vi "Draw Loops.vi"(7 "Action Diagram Sizing":T1, 10 "Action Diagram In":picture, 11 "Actions":T2={"Init"=FALSE, "Start"=FALSE, "Run"=TRUE, "Stop"=FALSE, "Close"=FALSE}) -> (2 "Action Diagram":picture)   [LabVIEW 2022 SP3, in "FlexBlocks Support.lvlib"]
uses:
  FlexBlocks Support.lvlib
  Action Selections.ctl
  Action Diagram Sizing.ctl
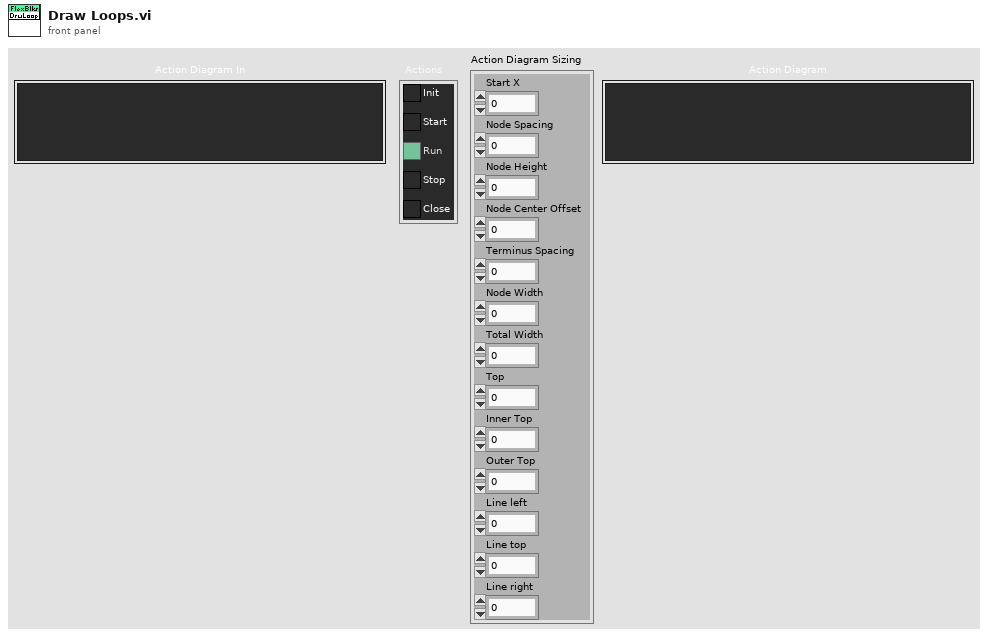
[diagram p1: front panel]
types:
  T1 = typedef "FlexBlocks Support.lvlib/Action Diagram Sizing.ctl" = cluster{"Start X":i32, "Node Spacing":i32, "Node Height":i32, "Node Center Offset":i32, "Terminus Spacing":i32, "Node Width":i32, "Total Width":i32, "Top":i32, "Inner Top":i32, "Outer Top":i32, "Line left":i32, "Line top":i32, "Line right":i32}
  T2 = typedef "FlexBlocks Support.lvlib/Action Selections.ctl" = cluster{"Init":bool, "Start":bool, "Run":bool, "Stop":bool, "Close":bool}
  T3 = cluster{"left":i16, "top":i16, "right":i16, "bottom":i16}
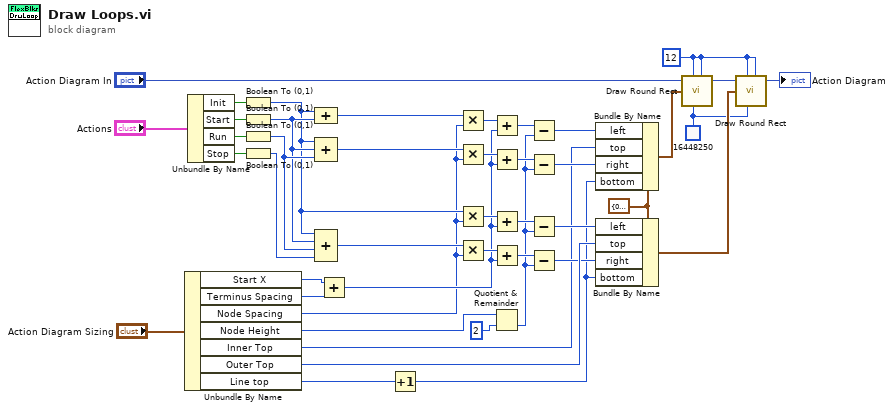
[diagram p0: block diagram]
diagram:
  w12 = T3 {"left"=0, "top"=0, "right"=0, "bottom"=0} ("rect")
  w10 = u32 16448250 ("color(black)")
  w17 = i16 12 ("oval width")
  n1 = Unbundle By Name("Action Diagram Sizing") -> ("Start X"=w31:i32, "Terminus Spacing"=w30:i32, "Node Spacing"=w1:i32, "Node Height"=w29:i32, "Inner Top"=w5:i32, "Outer Top"=w34:i32, "Line top"=w33:i32)
  n2 = Unbundle By Name("Actions") -> ("Init"=w42:bool, "Start"=w41:bool, "Run"=w40:bool, "Stop"=w39:bool)
  n3 = Boolean To (0,1)(Boolean=w42) -> (0, 1=w15:i16)
  n4 = Boolean To (0,1)(Boolean=w41) -> (0, 1=w25:i16)
  n5 = Boolean To (0,1)(Boolean=w40) -> (0, 1=w26:i16)
  n6 = Boolean To (0,1)(Boolean=w39) -> (0, 1=w38:i16)
  n7 = Compound Arithmetic op=ADD(w15, w25) -> (w19:i16)
  n8 = Compound Arithmetic op=ADD(w15, w25, w26) -> (w20:i16)
  n9 = Compound Arithmetic op=ADD(w15, w25, w26, w38) -> (w16:i16)
  n10 = Add(x=w31, y=w30) -> (x+y=w2:i32)
  n11 = Increment(x=w33) -> (x+1=w4:i32)
  n12 = Multiply(x=w19, y=w1) -> (x*y=w22:i32)
  n13 = Multiply(x=w20, y=w1) -> (x*y=w21:i32)
  n14 = Multiply(x=w15, y=w1) -> (x*y=w36:i32)
  n15 = Multiply(x=w16, y=w1) -> (x*y=w37:i32)
  n16 = Add(x=w22, y=w2) -> (x+y=w24:i32)
  n17 = Add(x=w21, y=w2) -> (x+y=w23:i32)
  n18 = Add(x=w36, y=w2) -> (x+y=w27:i32)
  n19 = Add(x=w37, y=w2) -> (x+y=w28:i32)
  n20 = Quotient & Remainder(x=w29, y=2) -> (floor(x/y)=w3:i32)  [unwired: 1 out]
  n21 = Subtract(x=w24, y=w3) -> (x-y=w7:i32)
  n22 = Subtract(x=w23, y=w3) -> (x-y=w6:i32)
  n23 = Subtract(x=w27, y=w3) -> (x-y=w14:i32)
  n24 = Subtract(x=w28, y=w3) -> (x-y=w13:i32)
  n25 = Bundle By Name(cluster=w12, "left"=w7, "top"=w5, "right"=w6, "bottom"=w4) -> (w9:T3)
  n26 = Bundle By Name(cluster=w12, "left"=w14, "top"=w34, "right"=w13, "bottom"=w4) -> (w11:T3)
  n27 = call <vilib>:"Draw Round Rect.vi"("picture"="Action Diagram In", "oval width"=w17, "rect"=w9, "color(black)"=w10, "oval height"=w17) -> ("new picture"=w18:picture)  [unwired: 4 in]
  n28 = call <vilib>:"Draw Round Rect.vi"("picture"=w18, "oval width"=w17, "rect"=w11, "color(black)"=w10, "oval height"=w17) -> ("new picture"=→"Action Diagram":picture)  [unwired: 4 in]
